vi "Write Data file name.vi"(1 "Data file name.":string) -> (0 "PASS/FAIL.":bool)   [LabVIEW 2010]
panel:
  # "Inputs:"
  # "Outputs."
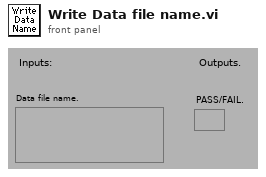
[diagram p1: front panel]
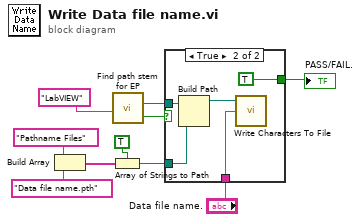
[diagram p0: block diagram]
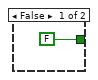
[diagram p2: hidden frame]
diagram:
  n1 = Build Array("Pathname Files", "Data file name.pth") -> (w7:string[])
  n2 = Array of Strings to Path(0:w7, 1:TRUE) -> (2:w10:path)
  n3 = call "Find path stem for EP.vi"("Node of path stem."="LabVIEW") -> ("Path stem."=w8:path, "PASS/FAIL"=w9:bool)
  n4 = case shown="True" w9 {
    tunnel: w8 -> [_ w16]
    tunnel: w10 -> [_ w15]
    tunnel: [FALSE TRUE] -> w2
    tunnel: "Data file name." -> [_ w12]
    frame False {
    }
    frame True {
      n5 = Build Path(base path=w16, name or relative path=w15) -> (appended path=w13:path)
      n6 = call <vilib>:"Write Characters To File.vi"("character string"=w12, "file path (dialog if empty)"=w13) -> ()  [unwired: 1 in, 3 out]
    }
  }
  "PASS/FAIL." <- w2
